vi "SubVI_SpikeCount.vi"(1 "Spike index input":i32[](array[numeric])) -> (0 "Total # spikes":i32)   [LabVIEW 2018]
panel:
  out "visualize spikes index":cluster{"Spike index input":i32[], i32[]}(graph)
  out "Firing rate vs spike index":cluster{"Spike index input":i32[], dbl[]}(graph)
  out "Spikes index":i32[](graph)
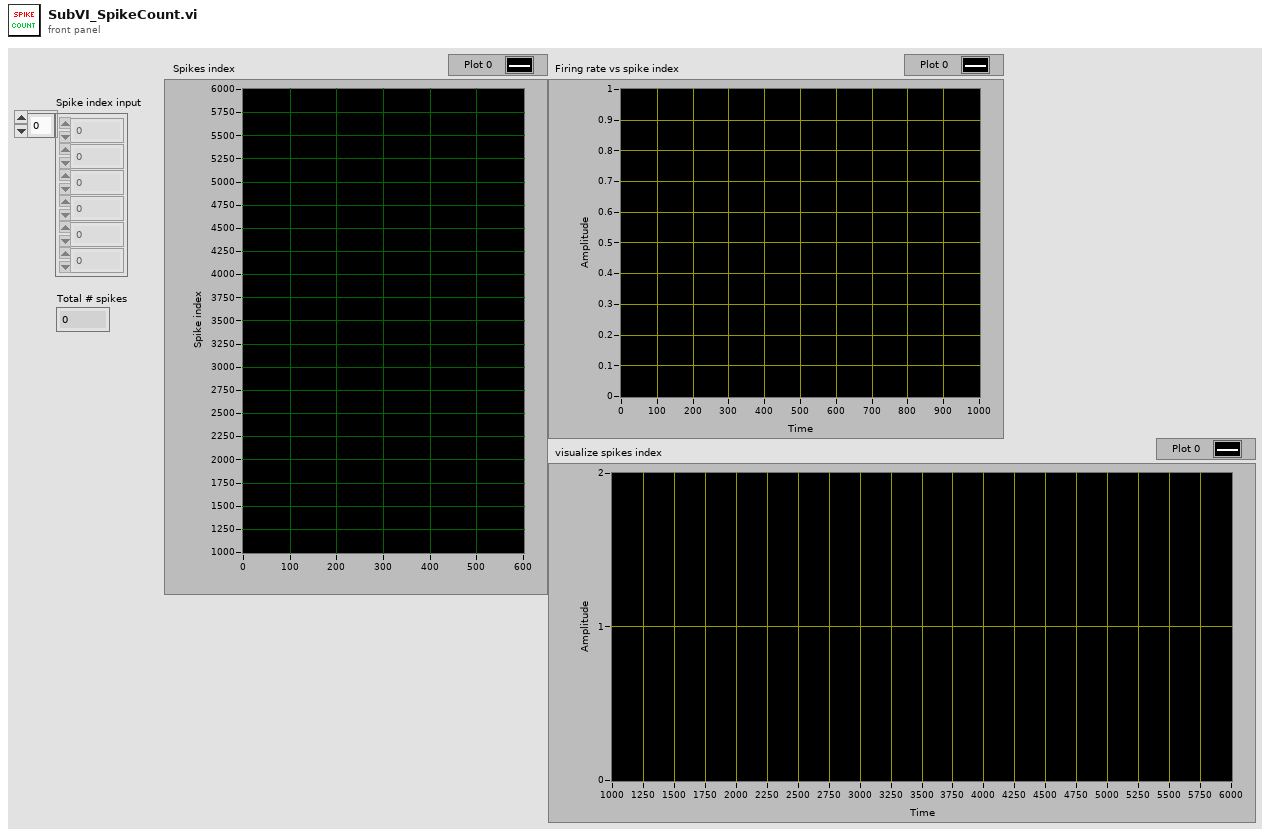
[diagram p1: front panel]
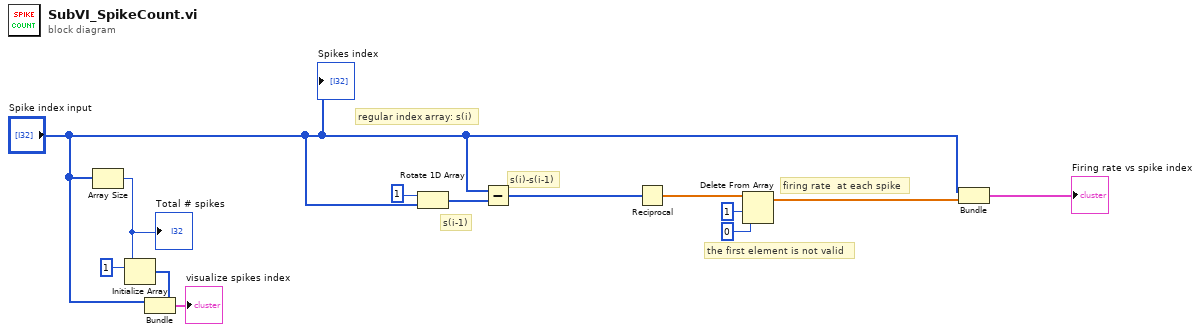
[diagram p0: block diagram]
diagram:
  # "firing rate  at each spike"
  # "the first element is not valid"
  # "s(i)-s(i-1)"
  # "s(i-1)"
  # "regular index array: s(i)"
  n1 = Array Size(array="Spike index input") -> (size(s)=w5:i32)
  "Total # spikes" <- w5
  n2 = Initialize Array(1 ("element"), w5) -> (w3:i32[])
  n3 = Bundle("Spike index input"="Spike index input", w3) -> (→"visualize spikes index":cluster{"Spike index input":i32[], i32[]})  [unwired: 1 in]
  n4 = Rotate 1D Array(1:"Spike index input", 2:1 ("n")) -> (0:w12:i32[])
  n5 = Subtract(x="Spike index input", y=w12) -> (x-y=w7:i32[])
  n6 = Reciprocal(x=w7) -> (1/x=w2:dbl[])
  n7 = Delete From Array(array=w2, length=1, index=0) -> (array with subset deleted=w8:dbl[])  [unwired: 1 out]
  n8 = Bundle("Spike index input"="Spike index input", w8) -> (→"Firing rate vs spike index":cluster{"Spike index input":i32[], dbl[]})  [unwired: 1 in]
  "Spikes index" <- "Spike index input"
